vi "find_files_in_paths.vi"(0 "TopLevelDataFilePath":path, 1 "File2Find":path, 2 "Item Name":string, 3 "Message Prefix":string, 4 "What to do string/file prompt":string, 6 "PromptFormissingFile":bool) -> (5 "Path":path, 7 "Relative Path to file":path)   [LabVIEW 2011]
doc: "Vi attempts to find the files even if the absolute file path is recorded correct. It will search a logical downstream file path to find the file set. This can be useful when files directory are copied from one location or one machine to another.\n\nStarts by checking if a path is entered."
panel:
  out "file or folder exists?":bool
  out "appended path":path
  out "error out":errorcluster
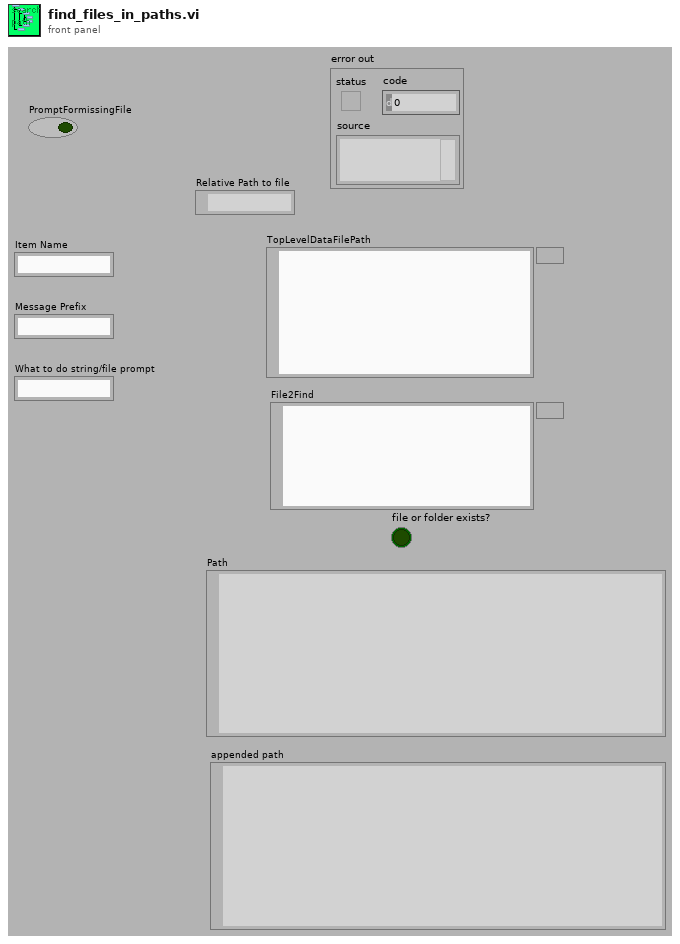
[diagram p1: front panel]
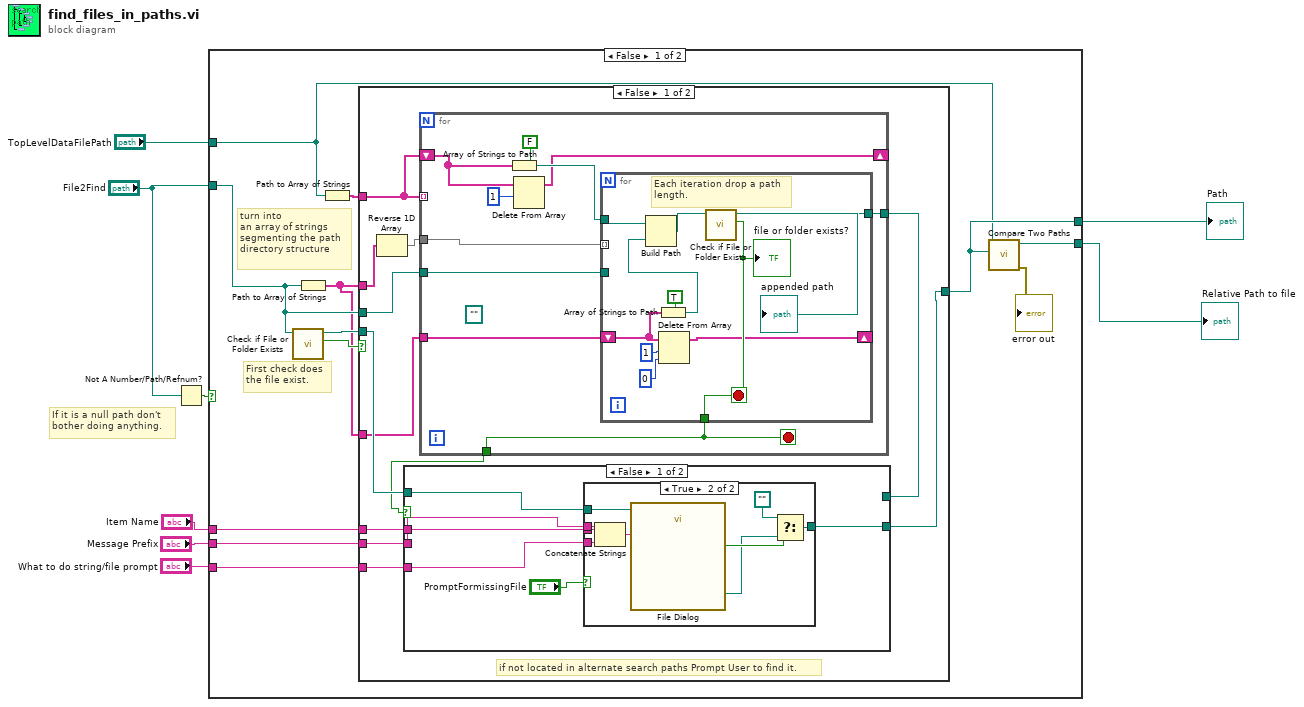
[diagram p0: block diagram]
diagram:
  # "If it is a null path don't\nbother doing anything."
  n1 = Not A Number/Path/Refnum?(number/path/refnum="File2Find") -> (NaN/Path/Refnum?=w1:bool)
  n2 = case shown="False" w1 {
    tunnel: "What to do string/file prompt" -> [w20 _]
    tunnel: "Message Prefix" -> [w19 _]
    tunnel: [w18 w71] -> w6
    tunnel: [w17 w71] -> w5
    tunnel: "TopLevelDataFilePath" -> [w16 _]
    tunnel: "Item Name" -> [w15 _]
    tunnel: "File2Find" -> [w10 w71]
    frame False {
      # "turn into\nan array of strings\nsegmenting the path\ndirectory structure"
      # "First check does\nthe file exist."
      n3 = call <vilib>:"Check if File or Folder Exists.vi"("path"=w10) -> ("file or folder exists?"=w12:bool, "dup path"=w13:path)  [unwired: 8 in, 1 out]
      n4 = Path to Array of Strings(0:w10) -> (2:w9:string[])  [unwired: 1 out]
      n5 = Path to Array of Strings(0:w16) -> (2:w14:string[])  [unwired: 1 out]
      n6 = case shown="False" w12 {
        tunnel: w13 -> [w28 w70]
        tunnel: [w29 w70] -> w18
        tunnel: w9 -> [w31 _]
        tunnel: w14 -> [w21 _]
        tunnel: w15 -> [w27 _]
        tunnel: w19 -> [w26 _]
        tunnel: w20 -> [w24 _]
        tunnel: w10 -> [w23 _]
        tunnel: w9 -> [w22 _]
        frame False {
          # "if not located in alternate search paths Prompt User to find it."
          n7 = Reverse 1D Array(array=w31) -> (reversed array=w32:string[])
          n8 = for {
            tunnel: w21 -> [_] mode=indexing
            tunnel: w32 -> [w59]
            tunnel: [w58] -> w30
            tunnel: [w57] -> w25
            tunnel: w23 -> [w56]
            tunnel: w22 -> [w55]
            shift-right: [w51] -> _
            shift-left: w21 -> [w50]
            stop <- w57 stop-if-true
            (unwired) path "" ("base path")
            n9 = Array of Strings to Path(0:w50, 1:FALSE ("relative")) -> (2:w52:path)
            n10 = Delete From Array(array=w50, length=1) -> (array with subset deleted=w51:string[])  [unwired: 1 in, 1 out]
            n11 = for {
              tunnel: w59 -> [_] mode=indexing
              tunnel: w52 -> [w66]
              tunnel: [w68] -> w58
              tunnel: [w67] -> w57
              tunnel: w56 -> [_]
              shift-right: [w63] -> _
              shift-left: w55 -> [w65]
              stop <- w67 stop-if-true
              # "Each iteration drop a path\nlength."
              n12 = Array of Strings to Path(0:w65, 1:TRUE ("relative")) -> (2:w61:path)
              n13 = Build Path(base path=w66, name or relative path=w61) -> (appended path=w69:path)
              "appended path" <- w69
              n14 = Delete From Array(array=w65, length=1, index=0) -> (array with subset deleted=w63:string[])  [unwired: 1 out]
              n15 = call <vilib>:"Check if File or Folder Exists.vi"("path"=w69) -> ("file or folder exists?"=w67:bool, "dup path"=w68:path)  [unwired: 8 in, 1 out]
              "file or folder exists?" <- w67
            }
          }
          n16 = case shown="False" w25 {
            tunnel: w30 -> [_ w49]
            tunnel: [w36 w49] -> w29
            tunnel: w28 -> [w38 _]
            tunnel: w27 -> [w37 _]
            tunnel: w26 -> [w35 _]
            tunnel: w24 -> [w34 _]
            frame False {
              n17 = case shown="True" "PromptFormissingFile" {
                tunnel: w38 -> [w39 w48]
                tunnel: w37 -> [_ w47]
                tunnel: [w39 w43] -> w36
                tunnel: w35 -> [_ w41]
                tunnel: w34 -> [_ w40]
                frame False {
                }
                frame True {
                  n18 = Concatenate Strings(w41, w47, w40) -> (w46:string)
                  n19 = call "File Dialog"("start path"=w48, "prompt"=w46) -> ("selected path"=w44:path, "cancelled"=w45:bool)  [unwired: 10 in, 2 out]
                  n20 = Select(t=path "", s=w45, f=w44) -> (s? t:f=w43:path)
                }
              }
            }
            frame True {
            }
          }
        }
        frame True {
          # "if the path exists as a complete path\nkeep the absolute path"
        }
      }
      n21 = call <vilib>:"Compare Two Paths.vi"("Path 2"=w18, "Path 1"=w16) -> ("error out"=→"error out":errorcluster, "Relative Path from 1 to 2"=w17:path)  [unwired: 6 in, 2 out]
    }
    frame True {
      # "don't both if it is NOT A PATH"
    }
  }
  "Path" <- w6
  "Relative Path to file" <- w5
